vi "deCOB-ID.vi"(0 "Cob ID":u32) -> (1 "Node ID":u16, 2 "Function code":T1 items=["NMT", "SYNC", "TIME STAMP", "EMERGENCY", "PDO1 (tx)", "PDO1 (rx)", "PDO2 (tx)", "PDO2 (rx)", "PDO3 (tx)", "PDO3 (rx)", "PDO4 (tx)", "PDO4 (rx)", "SDO (tx)", "SDO (rx)", "NMT Error Control"])   [LabVIEW 2017, in "canopen.lvlib" / "CANopen.lvclass"]
doc: "Decomposes a canonical COB-ID into its function code and node ID. This is the reverse operation of enCOB-ID."
uses:
  CANopen.lvclass
  FunctionCode.ctl
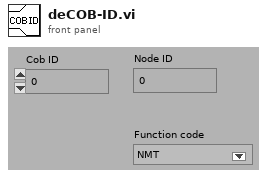
[diagram p1: front panel]
types:
  T1 = typedef "canopen.lvlib/CANopen.lvclass/FunctionCode.ctl" = u8
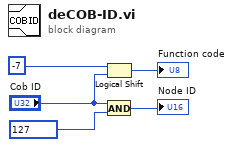
[diagram p0: block diagram]
diagram:
  n1 = Logical Shift(y=i16 -7, x="Cob ID") -> (x << y=→"Function code":u32)
  n2 = And(x="Cob ID", y=u32 127) -> (x .and. y?=→"Node ID":u32)
